vi "Read Characteristics file reference.vi"(8 "error in (no error)":errorcluster, 11 "Analysis params in":refnum<class "CV-Analysis.lvclass">) -> (0 "error out":errorcluster, 2 "Characteristics file reference":refnum<k34>, 3 "Analysis params out":refnum<class "CV-Analysis.lvclass">)   [LabVIEW 2013, in "CameraVision.lvlib" / "CV-Analysis.lvclass"]
uses:
  CV-Analysis.lvclass
  CV-Analysis.lvclass/CV-Analysis.ctl
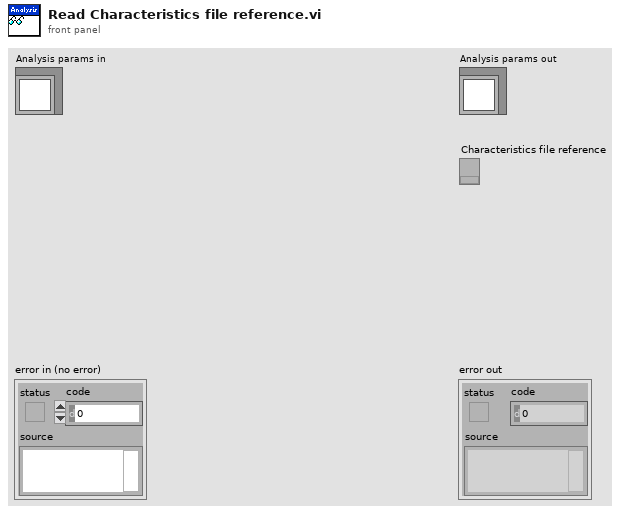
[diagram p1: front panel]
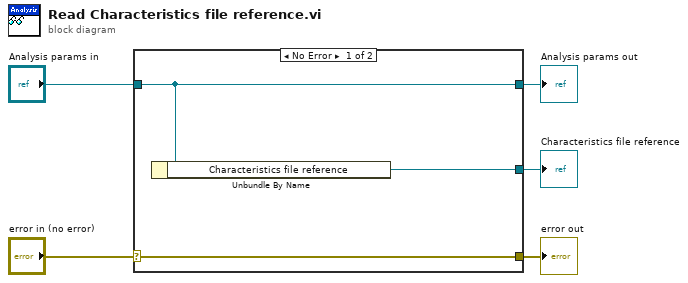
[diagram p0: block diagram]
diagram:
  n1 = case shown="No Error" "error in (no error)" {
    selector: "error in (no error)" -> [w8 w9]
    tunnel: [w8 w9] -> w4
    tunnel: [w7 w10] -> w2
    tunnel: "Analysis params in" -> [w7 w10]
    tunnel: [w6 _] -> w1
    frame No Error {
      n2 = Unbundle By Name(w7) -> ("Characteristics file reference"=w6:refnum<k34>)
    }
    frame Error {
    }
  }
  "error out" <- w4
  "Analysis params out" <- w2
  "Characteristics file reference" <- w1
